vi "Test XYZ Table Stage Module.vi"() -> ()   [LabVIEW 2018]
uses:
  General/Controls/Set Get Controls.ctl
  Hardware Mfg/Thorlabs Translation Stages/Controls/Motion Translation Module Control.ctl
  General/Controls/Translation Stage Types.ctl
  Hardware Mfg/Thorlabs Translation Stages/Controls/Translation Stage Cluster.ctl
  General/Controls/Translation Stage Parameters.ctl
panel:
  in  "waitTimeout (ms)":i32
  in  "Velocity":dbl
  in  "Acceleration":dbl
  in  "VelocityMaximum":dbl caption="Max Velocity"
  in  "AccelerationMaximum":dbl caption="Max Acceleration"
  in  "Position 2":dbl caption="Position"
  in  "Axis":enum16{"X Axis", "Y Axis", "Z Axis"}(ring)
  out "Error Out":errorcluster
  in  "Uninit":bool
  in  "Init":bool
  in  "Cancel Button":bool
  in  "Position":bool
  in  "Stop":bool
  in  "Home":bool
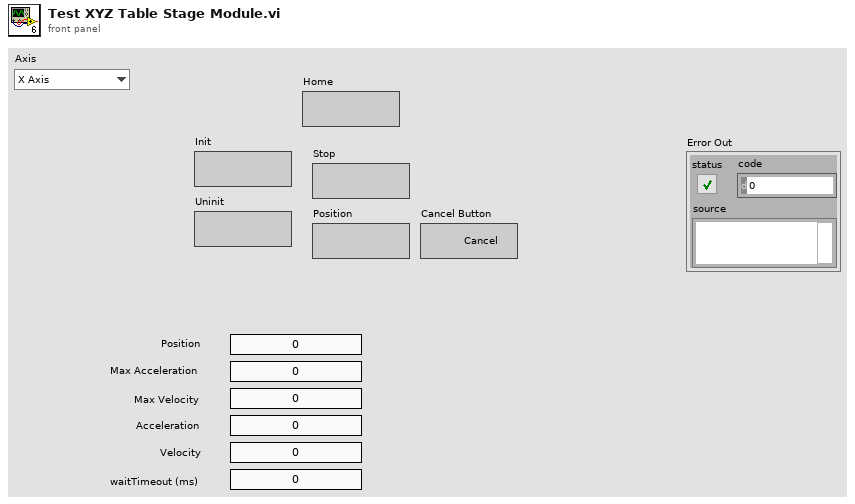
[diagram p1: front panel]
types:
  T1 = typedef "Translation Stage Parameters.ctl" = cluster{"X Stage":T2, "Y Stage":T2, "Z Stage":T2}
  T2 = typedef "Translation Stage Cluster.ctl" = cluster{"Position":dbl, "Is.Enabled?":bool, "Is.Connected?":bool, "Device SN":string, "AccelerationMaximum":dbl, "VelocityMaximum":dbl, "Acceleration":dbl, "Velocity":dbl, "waitTimeout (ms)":i32, "Model":T3, "Is.Homed?":bool}
  T3 = typedef "Translation Stage Types.ctl" = enum16{"None", "Thorlabs LTS", "Thorlabs MLJ"}
  T4 = typedef "Motion Translation Module Control.ctl" = enum16{"Init", "Home", "Status", "Velocity/Accel", "Position", "Jog", "Stop", "Uninit", "Enable", "Disable"}
  T5 = typedef "Set Get Controls.ctl" = enum16{"Set", "Get"}
  T6 = typedef "System Parameters.ctl" = cluster{"Optical Parameters":T7, "Vibratome":T8, "Table Stages":T1, "Imaging Parameter":T9, "Galvo HW Parameters":cluster{"Analog Out Channel":tag, "Min Voltage":dbl, "Max Voltage":dbl, "Pixel Clock Source":tag, "Sample Rate":dbl, "Line Clock Out Ch":tag}, "Alazar parameters":T11}
  T7 = typedef "Optical Parameters.ctl" = cluster{"Obj. Focal Length [mm]":dbl, "Scan Lens EFL[mm]":dbl, "Tube Lens EFL[mm]":dbl, "Galvo V Range (+/-)":dbl, "Galvo Max Half Angle [Deg]":dbl, "Max Galvo Range[%]":dbl}
  T8 = typedef "Vibratome Parameters.ctl" = cluster{"Z Bottom [mm]":dbl, "Pre Cut Dwell [s]":dbl, "Blade Frequency [RPM]":u16, "Slice Speed [mm/s]":dbl, "Post Cut Dwell [s]":dbl, "Ramp Time [s]":dbl, "Start X [mm]":dbl, "Start Y [mm]":dbl, "Slice Length [mm]":dbl, "Slice Axis":enum16{"X Axis", "Y Axis", "Z Axis"}, "Controller VISA Ref":refnum<visa-resource-name>}
  T9 = typedef "Imaging Parameters.ctl" = cluster{"Raster Scan Direction":T10, "Pixel Dwell Time [Clock Cycles]":u16, "Flyback Time [Clock Cycles]":u16, "XY Center [um]":cluster{"X":dbl, "Y":dbl}, "Pixel Step Size [um]":dbl, "XY Image Size":enum16{"32 x 32", "64 x 64", "128 x 128", "256 x 256", "512 x 512", "1024 x 1024", "2048 x 2048"}, "Custom":bool, "Custom Size":cluster{"X":u16, "Y":u16}, "Line Averages":u8}
  T10 = typedef "Scan Direction.ctl" = enum16{"Uni Directional", "Bi Directional", "None"}
  T11 = typedef "Alazar parameters.ctl" = cluster{"Trigger Settings":cluster{"General Trigger Settings":T12, "Trigger Engine 1":T13, "Trigger Engine 2":T13}, "Capture Clock":T14, "Device ID":T15, "Ch A Input Control":T16, "Ch B Input Control":T16, "Acq Settings":T17, "Cluster":T18}
  T12 = typedef "General Trigger Settings.ctl" = cluster{"Trigger Operation":u32, "Coupling ID":u32, "Range ID":u32, "Delay":u32, "Timeout Ticks":u32, "Mode":u32, "Parameter":u32}
  T13 = typedef "Trigger Engine Controls.ctl" = cluster{"Trigger Engine":u32, "Source":u32, "Slope":u32, "Level":u32}
  T14 = typedef "Clock Controls.ctl" = cluster{"Sample Rate":u32, "Decimation":u32, "Source":u32, "Edge":u32}
  T15 = typedef "Alazar Device ID.ctl" = cluster{"System ID":u32, "Board ID":u32}
  T16 = typedef "Channel Input Controls.ctl" = cluster{"Channel":u8, "Coupling":u32, "Range":u32, "Impedance":u32}
  T17 = typedef "Alazar Acquisition Settings.ctl" = cluster{"Window Type":u32, "Record Length":u32, "Footer":u32, "Output Format":u32, "Offset":u32, "Records Per Buffer":u32, "Samples per record":u32, "Records Count (Records/Acq)":u32}
  T18 = typedef "Control cluster.ctl" = cluster{"FFT value magnification":dbl, "max queue size (-1, unlimited)":i32, "File Type":T19, "file path":path, "#A-lines to save":u32, "#Z pixels to save":u32, "ImageDescription":string, "Convert to U16?":bool}
  T19 = typedef "file type.ctl" = enum16{"text", "Tiff", "binary"}
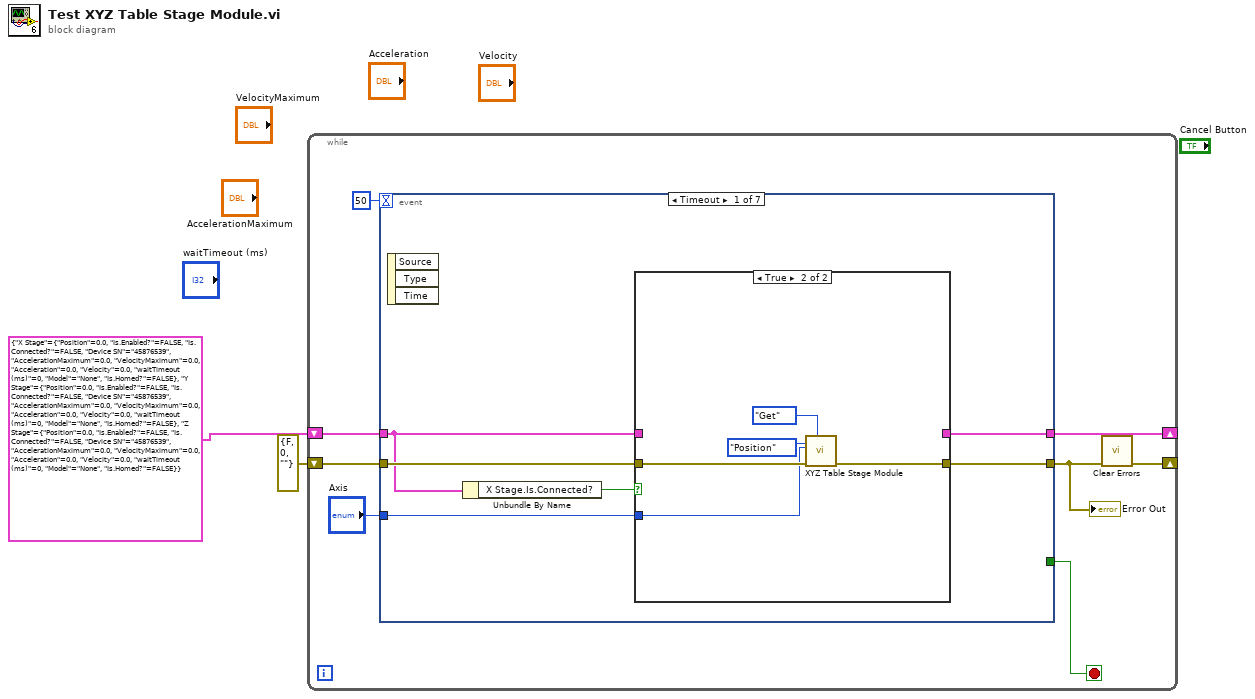
[diagram p0: block diagram]
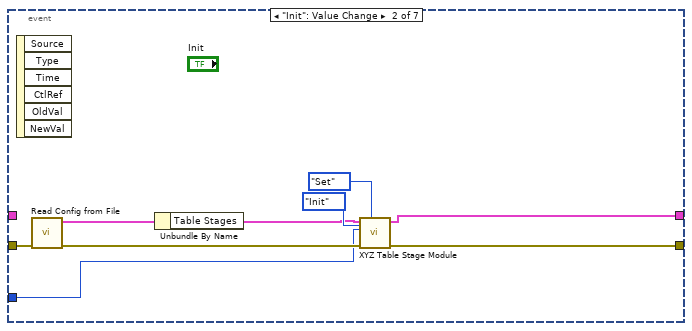
[diagram p3: hidden frame]
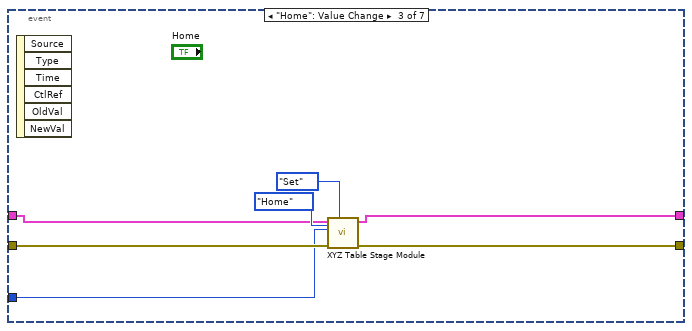
[diagram p4: hidden frame]
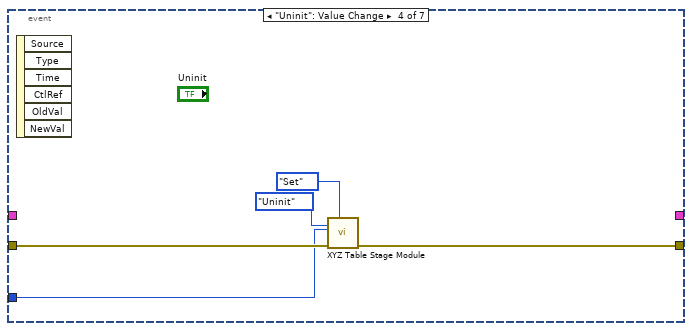
[diagram p5: hidden frame]
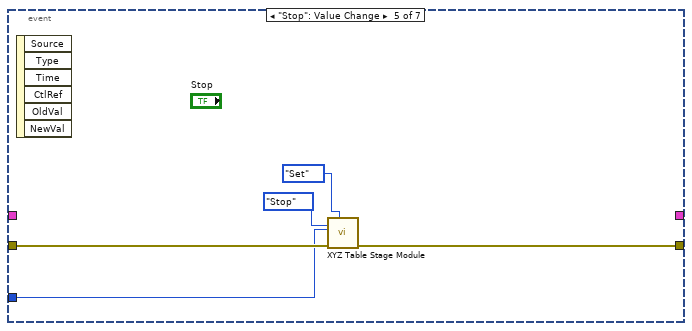
[diagram p6: hidden frame]
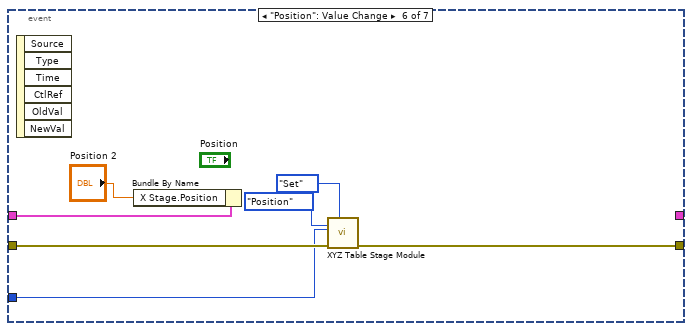
[diagram p7: hidden frame]
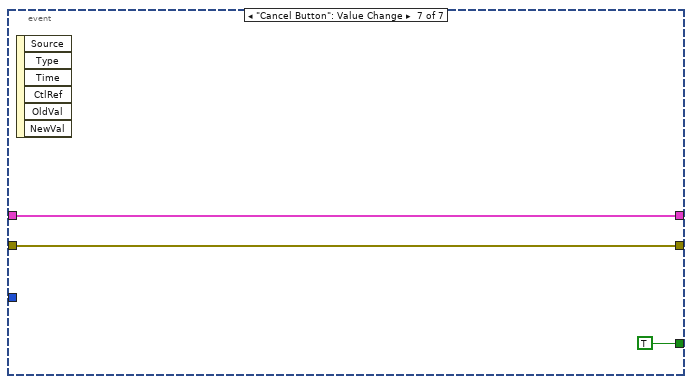
[diagram p8: hidden frame]
diagram:
  n1 = while {
    shift-right: [w3] -> _
    shift-left: errorcluster {"status"=FALSE, "code"=0, "source"=""} ("Error Out") -> [w7]
    shift-right: [w5] -> _
    shift-left: T1 {"X Stage"={"Position"=0.0, "Is.Enabled?"=FALSE, "Is.Connected?"=FALSE, "Device SN"="45876539", "AccelerationMaximum"=0.0, "VelocityMaximum"=0.0, "Acceleration"=0.0, "Velocity"=0.0, "waitTimeout (ms)"=0, "Model"=enum."None", "Is.Homed?"=FALSE}, "Y Stage"={"Position"=0.0, "Is.Enabled?"=FALSE, "Is.Connected?"=FALSE, "Device SN"="45876539", "AccelerationMaximum"=0.0, "VelocityMaximum"=0.0, "Acceleration"=0.0, "Velocity"=0.0, "waitTimeout (ms)"=0, "Model"=enum."None", "Is.Homed?"=FALSE}, "Z Stage"={"Position"=0.0, "Is.Enabled?"=FALSE, "Is.Connected?"=FALSE, "Device SN"="45876539", "AccelerationMaximum"=0.0, "VelocityMaximum"=0.0, "Acceleration"=0.0, "Velocity"=0.0, "waitTimeout (ms)"=0, "Model"=enum."None", "Is.Homed?"=FALSE}} ("Table Stages") -> [w6]
    stop <- w9 stop-if-true
    n2 = event shown="[0] Timeout" {
      selector: _ -> [_ _ _ _ _ _ _]
      dyn-events: _ -> [_ _ _ _ _ _ _]
      timeout: 50 -> [_ _ _ _ _ _ _]
      tunnel: [_ _ _ _ _ _ TRUE] -> w9
      tunnel: [w16 w24 w33 _ _ _ w58] -> w5
      tunnel: w6 -> [w13 _ w34 _ _ w52 w58]
      tunnel: [w15 w32 w38 w43 w48 w55 w57] -> w8
      tunnel: w7 -> [w14 w29 w39 w44 w49 w56 w57]
      tunnel: "Axis" -> [w11 w27 w35 w40 w45 w50 _]
      event Timeout {
        n3 = event-data() -> ()  [unwired: 1 in, 3 out]
        n4 = Unbundle By Name(w13) -> ("X Stage.Is.Connected?"=w12:bool)
        n5 = case shown="True" w12 {
          tunnel: [w18 _] -> w16
          tunnel: [w17 w21] -> w15
          tunnel: w14 -> [w17 w20]
          tunnel: w13 -> [w18 _]
          tunnel: w11 -> [_ w19]
          frame False {
          }
          frame True {
            n6 = call "XYZ Table Stage Module.vi"("Set/Get"=Set_Get_Controls."Get", "Action"=Motion_Translation_Module_Control."Position", "Error In"=w20, "Axis"=w19) -> ("Error Out"=w21:errorcluster)  [unwired: 6 in, 1 out]
          }
        }
      }
      event "Init": Value Change {
        n7 = event-data() -> ()  [unwired: 1 in, 6 out]
        n8 = call "Read Config from File.vi"("error in (no error)"=w29) -> ("error out"=w28:errorcluster, "System Parameters"=w26:T6)  [unwired: 9 in]
        n9 = Unbundle By Name(w26) -> ("Table Stages"=w25:T1)
        n10 = call "XYZ Table Stage Module.vi"("Set/Get"=Set_Get_Controls."Set", "Action"=Motion_Translation_Module_Control."Init", "Error In"=w28, "Axis"=w27, "Table Stages"=w25) -> ("Error Out"=w32:errorcluster, "Table Stages [out]"=w24:T1)  [unwired: 5 in]
      }
      event "Home": Value Change {
        n11 = event-data() -> ()  [unwired: 1 in, 6 out]
        n12 = call "XYZ Table Stage Module.vi"("Set/Get"=Set_Get_Controls."Set", "Action"=Motion_Translation_Module_Control."Home", "Error In"=w39, "Axis"=w35, "Table Stages"=w34) -> ("Error Out"=w38:errorcluster, "Table Stages [out]"=w33:T1)  [unwired: 5 in]
      }
      event "Uninit": Value Change {
        n13 = event-data() -> ()  [unwired: 1 in, 6 out]
        n14 = call "XYZ Table Stage Module.vi"("Set/Get"=Set_Get_Controls."Set", "Action"=Motion_Translation_Module_Control."Uninit", "Error In"=w44, "Axis"=w40) -> ("Error Out"=w43:errorcluster)  [unwired: 6 in, 1 out]
      }
      event "Stop": Value Change {
        n15 = event-data() -> ()  [unwired: 1 in, 6 out]
        n16 = call "XYZ Table Stage Module.vi"("Set/Get"=Set_Get_Controls."Set", "Action"=Motion_Translation_Module_Control."Stop", "Error In"=w49, "Axis"=w45) -> ("Error Out"=w48:errorcluster)  [unwired: 6 in, 1 out]
      }
      event "Position": Value Change {
        n17 = event-data() -> ()  [unwired: 1 in, 6 out]
        n18 = Bundle By Name(cluster=w52, "X Stage.Position"="Position 2") -> ()  [unwired: 1 out]
        n19 = call "XYZ Table Stage Module.vi"("Set/Get"=Set_Get_Controls."Set", "Action"=Motion_Translation_Module_Control."Position", "Error In"=w56, "Axis"=w50) -> ("Error Out"=w55:errorcluster)  [unwired: 6 in, 1 out]
      }
      event "Cancel Button": Value Change {
        n20 = event-data() -> ()  [unwired: 1 in, 6 out]
      }
    }
    "Error Out" <- w8
    n21 = call <vilib>:"Clear Errors.vi"("error in (no error)"=w8) -> ("error out"=w3:errorcluster)  [unwired: 5 in, 1 out]
  }
